vi "AI Channels--constant.vi"() -> (3 "AI Channels":tag[](array[tag])=["A/AI0", "A/AI1", "A/AI2", "A/AI3", "B/AI0", "B/AI1", "B/AI2", "B/AI3", "C/AI0", "C/AI1"])   [LabVIEW 2021, in "Common Files.lvlib"]
uses:
  Common Files.lvlib
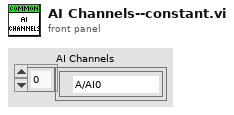
[diagram p1: front panel]
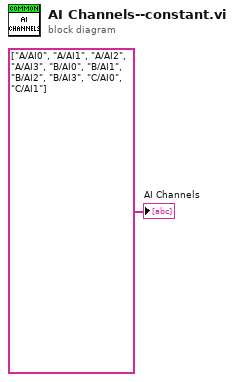
[diagram p0: block diagram]
diagram:
  "AI Channels" <- tag[] ["A/AI0", "A/AI1", "A/AI2", "A/AI3", "B/AI0", "B/AI1", "B/AI2", "B/AI3", "C/AI0", "C/AI1"] ("Channel Names")
